vi "DAQ Read.vi"(6 "Virtual Dev Error (F)":bool, 8 "error in (no error)":errorcluster, 11 "Refs Data in":T1) -> (0 "error out":errorcluster, 2 "Data":dbl, 3 "Refs Data out":T1)   [LabVIEW 2013]
doc: "Odcztuje dane z wybranego wejœcia analogowego karty rzeczywistej\nlub symuluje pobór danej z karty wirtualnej"
uses:
  inne pliki/RefData.ctl
  inne pliki/DevSetUp.ctl
  <vilib>/DAQmx/read.llb/DAQmx Read (Analog DBL 1Chan 1Samp).vi
  <vilib>/DAQmx/miscellaneous.llb/DAQmx Fill In Error Info.vi
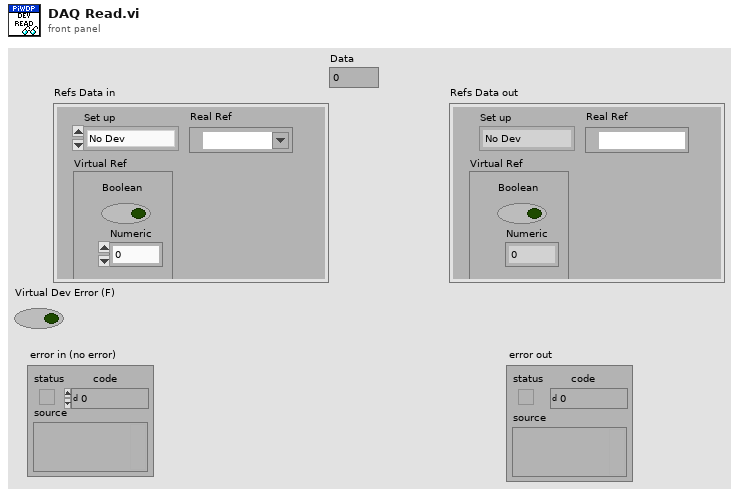
[diagram p1: front panel]
types:
  T1 = typedef "RefData.ctl" = cluster{"Virtual Ref":cluster{"Numeric":dbl, "Boolean":bool}, "Real Ref":refnum<k21>, "Set up":T2}
  T2 = typedef "DevSetUp.ctl" = enum16{"No Dev", "Virtual Dev", "Real Dev"}
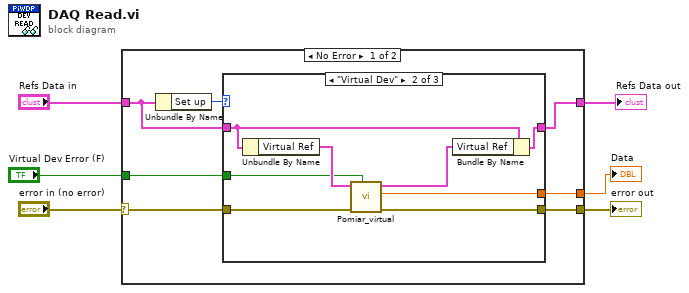
[diagram p0: block diagram]
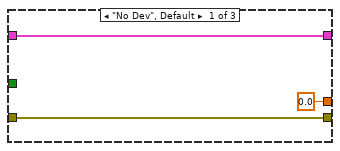
[diagram p2: hidden frame]
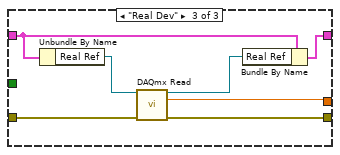
[diagram p3: hidden frame]
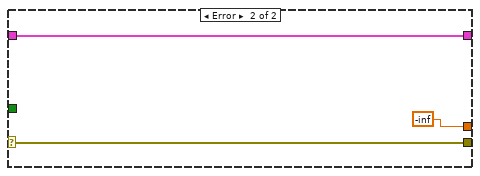
[diagram p4: hidden frame]
diagram:
  n1 = case shown="No Error" "error in (no error)" {
    selector: "error in (no error)" -> [w12 w34]
    tunnel: [w11 w34] -> w5
    tunnel: "Refs Data in" -> [w9 w32]
    tunnel: [w10 -inf] -> w3
    tunnel: [w8 w32] -> w2
    tunnel: "Virtual Dev Error (F)" -> [w7 _]
    frame No Error {
      n2 = Unbundle By Name(w9) -> ("Set up"=w13:T2)
      n3 = case shown="\"Virtual Dev\"" w13 {
        tunnel: w12 -> [w15 w24 w31]
        tunnel: [w15 w23 w30] -> w11
        tunnel: [0.0 ("out") w22 w29] -> w10
        tunnel: w9 -> [w16 w20 w28]
        tunnel: [w16 w18 w27] -> w8
        tunnel: w7 -> [_ w17 _]
        frame "No Dev", Default {
        }
        frame "Virtual Dev" {
          n4 = Unbundle By Name(w20) -> ("Virtual Ref"=w21:cluster{"Numeric":dbl, "Boolean":bool})
          n5 = call "Pomiar_virtual.vi"("Error Generate"=w17, "error in (no error)"=w24, "Reference in"=w21) -> ("error out"=w23:errorcluster, "out"=w22:dbl, "Reference out"=w19:cluster{"Numeric":dbl, "Boolean":bool})  [unwired: 6 in]
          n6 = Bundle By Name(cluster=w20, "Virtual Ref"=w19) -> (w18:T1)
        }
        frame "Real Dev" {
          n7 = Unbundle By Name(w28) -> ("Real Ref"=w26:refnum<k21>)
          n8 = call-poly <vilib>:"DAQmx Read.vi"("task/channels in"=w26, "error in"=w31) -> ("task out"=w25:refnum<k21>, "data"=w29:dbl, "error out"=w30:errorcluster)  [unwired: 11 in]
          n9 = Bundle By Name(cluster=w28, "Real Ref"=w25) -> (w27:T1)
        }
      }
    }
    frame Error {
    }
  }
  "error out" <- w5
  "Refs Data out" <- w2
  "Data" <- w3
